vi "Launch Event Handlers.vi"(8 "error in (no error)":errorcluster, 11 "IEventAggregator In":refnum<class "IEventAggregator.lvclass">) -> (0 "error out":errorcluster, 3 "IEventAggregator Out":refnum<class "IEventAggregator.lvclass">)   [LabVIEW 2017, in "ActorEvents.lvlib" / "IEventAggregator.lvclass"]
uses:
  IEventAggregator.lvclass
  C:/Program Files (x86)/National Instruments/LabVIEW 2017/vi.lib/ActorFramework/Actor/Actor.lvclass
  IEventAggregator.lvclass/IEventAggregator.ctl
  IEventHandler/IEventHandler.lvclass
  <vilib>/ActorFramework/Actor/Actor.lvclass/Actor.ctl
  <vilib>/ActorFramework/Message Enqueuer/Message Enqueuer.lvclass/Message Enqueuer.ctl
  IEventHandler/IEventHandler.lvclass/IEventHandler.ctl
  <vilib>/ActorFramework/Actor/Read Self Enqueuer.vi
  <vilib>/ActorFramework/Message Enqueuer/Init from Existing Queue.vi
  <vilib>/ActorFramework/Actor/Launch Nested Actor.vi
  <vilib>/ActorFramework/Message Enqueuer/Message Enqueuer.lvclass
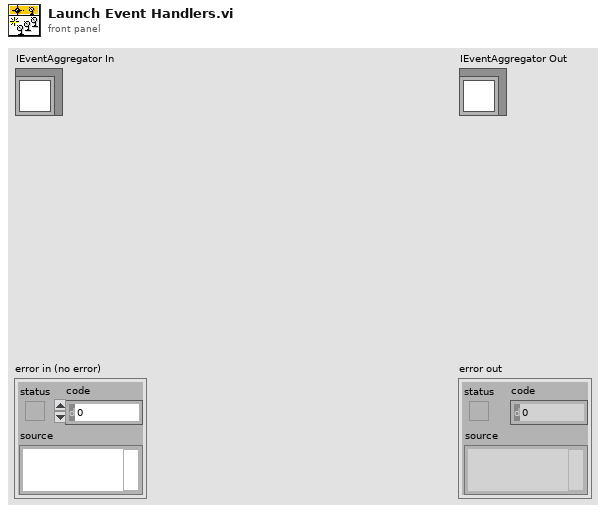
[diagram p1: front panel]
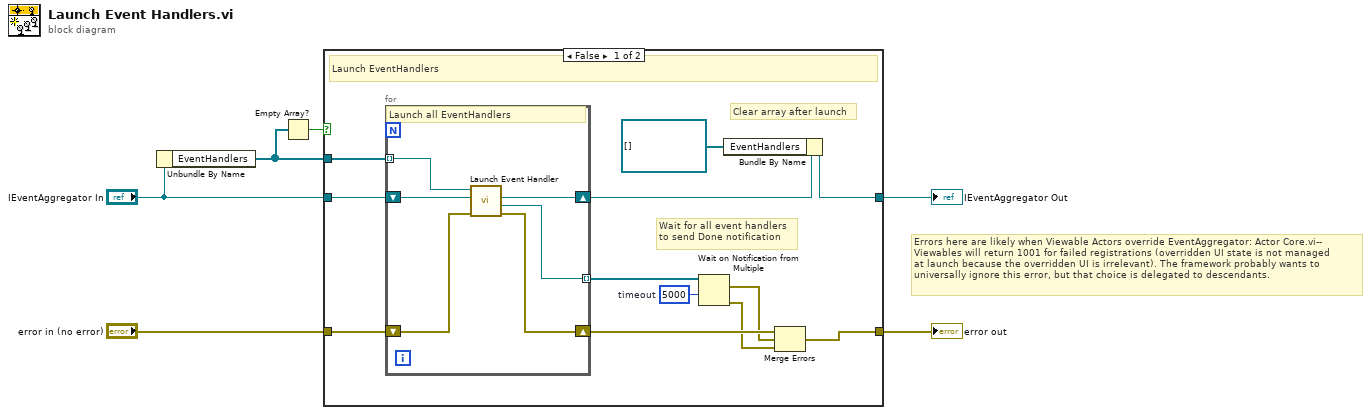
[diagram p0: block diagram]
diagram:
  # "Errors here are likely when Viewable Actors override EventAggregator: Actor Core.vi--\nViewables will return 1001 for failed registrations (overridden UI state is not managed\nat launch because the overridden UI is irrelevant). The framework probably wants to\nuniversally ignore this error, but that choice is delegated to descendants."
  n1 = Unbundle By Name("IEventAggregator In") -> ("EventHandlers"=w1:refnum<class "IEventHandler.lvclass">[])
  n2 = Empty Array?(array=w1) -> (empty?=w2:bool)
  n3 = case shown="False" w2 {
    tunnel: "error in (no error)" -> [w16 w25]
    tunnel: [w14 w25] -> w5
    tunnel: "IEventAggregator In" -> [w13 w26]
    tunnel: w1 -> [w12 _]
    tunnel: [w11 w26] -> w3
    frame False {
      w15 = 5000  # timeout
      # "Clear array after launch"
      # "Wait for all event handlers\nto send Done notification"
      # "Launch EventHandlers"
      n4 = for {
        shift-right: [w23] -> w18
        shift-left: w13 -> [w24]
        tunnel: w12 -> [w22] mode=indexing
        tunnel: [w21] -> w17 mode=indexing
        shift-right: [w19] -> w9
        shift-left: w16 -> [w20]
        # "Launch all EventHandlers"
        n5 = call "Launch Event Handler.vi"("error in (no error)"=w20, "EventAggregator In"=w24, "EventHandler In"=w22) -> ("error out"=w19:errorcluster, "Registration Done Notifier"=w21:refnum<notifier>, "EventAggregator Out"=w23:refnum<class "IEventAggregator.lvclass">)  [unwired: 5 in, 1 out]
      }
      n6 = Wait on Notification from Multiple(0:w17, 2:w15) -> (9:w8:errorcluster[], 11:w7:errorcluster)  [unwired: 2 in, 2 out]
      n7 = Bundle By Name(cluster=w18, "EventHandlers"=refnum<class "IEventHandler.lvclass">[] []) -> (w11:refnum<class "IEventAggregator.lvclass">)
      n8 = Merge Errors(w9, w8, w7) -> (w14:errorcluster)
    }
    frame True {
      # "Empty array -- No handlers to launch"
    }
  }
  "error out" <- w5
  "IEventAggregator Out" <- w3
